vi "Start Acquisition and Logging.vi"(8 "error in (no error)":errorcluster caption="错误输入（无错误）", 11 "Acquisition and Logging Configuration":T1={"Samples per Read"=100, "Number of Reads to Save"=20, "Number of Channels"=4, "Channel Scale Array"=[1.0, 1.0, 1.0, 1.0], "Channel Names"=["Mod1\\AI0", "Mod1\\AI1", "Mod1\\AI2", "Mod1\\AI3"], "Trigger - RMS Value"=0.9999999999999994, "Trigger - Channel"=0, "Trigger - Time (Minute)"=10, "TDMS Properties"=[], "Data File Name"="cRIO_Data", "Date Rate"=20} caption="采集与记录设置" {"Date Rate" items=["51.200 kS/s (NI 9234)"=1, "25.600 kS/s (NI 9234)"=2, "17.067 kS/s (NI 9234)"=3, "12.80 kS/s (NI 9234)"=4, "10.240 kS/s (NI 9234)"=5, "8.533 kS/s (NI 9234)"=6, "7.314 kS/s (NI 9234)"=7, "6.400 kS/s (NI 9234)"=8, "5.689 kS/s (NI 9234)"=9, "5.120 kS/s (NI 9234)"=10, "4.654 kS/s (NI 9234)"=11, "4.267 kS/s (NI 9234)"=12, "3.938 kS/s (NI 9234)"=13, "3.657 kS/s (NI 9234)"=14, "3.413 kS/s (NI 9234)"=15, "3.200 kS/s (NI 9234)"=16, "3.012 kS/s (NI 9234)"=17, "2.845 kS/s (NI 9234)"=18, "2.695 kS/s (NI 9234)"=19, "2.560 kS/s (NI 9234)"=20, "2.438 kS/s (NI 9234)"=21, "2.328 kS/s (NI 9234)"=22, "2.226 kS/s (NI 9234)"=23, "2.133 kS/s (NI 9234)"=24, "2.048 kS/s (NI 9234)"=25, "1.969 kS/s (NI 9234)"=26, "1.896 kS/s (NI 9234)"=27, "1.829 kS/s (NI 9234)"=28, "1.765 kS/s (NI 9234)"=29, "1.707 kS/s (NI 9234)"=30, "1.652 kS/s (NI 9234)"=31]}) -> (0 "error out":errorcluster caption="错误输出", 1 "Wait on IRQ Timeout?":bool caption="等待IRQ超时？", 2 "Total Buffer Size":i32 caption="全部缓冲区大小", 3 "FPGA VI Reference":T4 caption="FPGA VI引用")   [LabVIEW 2013]
uses:
  controls/FPGA VI Reference.ctl
  controls/Acquisition and Logging Configuration.ctl
  controls/TDMS Properties.ctl
  <vilib>/LabVIEW Targets/FPGA/cRIO/shared/nicrio_ModuleControls/nicrio_cRIO-9234_DataRatesRing2.ctl
  <vilib>/rvi/interface/common/niFpgaWaitOnOcc.vi
  <vilib>/FPGAPlugInAG/cRIO-9074/niLvFpga_Open_cRIO-9074.vi
  <vilib>/FPGAPlugInAG/cRIO-9074/niLvFpga_Reset_cRIO-9074.vi
  <vilib>/Utility/error.llb/Error Cluster From Error Code.vi
  <vilib>/rvi/errors/niLvFpgaAdjustHostInterfaceError.vi
  <vilib>/FPGAPlugInAG/cRIO-9074/niLvFpga_Run_cRIO-9074.vi
  <vilib>/RVI Host/nirviSupport.llb/nirviErrorClusterFromErrorCode.vi
  <vilib>/rvi/interface/nirviOpenFPGA/nirviOpenFPGA.xnode
  FPGA Bitfiles/LabVIEWFPGAWavef_FPGA_FPGAMain_vTbN89OLNVY.lvbitx
  FPGA Main.vi
  <vilib>/rvi/interface/nirviMethod/nirviMethod.xnode
  <vilib>/rvi/interface/nirviReadWriteControl/nirviReadWriteControl.xnode
  <vilib>/rvi/errors/niLvFpgaMergeErrorWithErrorCode.vi
  NiFpgaLv.dll
  <vilib>/FPGAPlugInAG/cRIO-9074/niLvFpga_ConfigureFifo_cRIO-9074.vi
  <vilib>/FPGAPlugInAG/cRIO-9074/niLvFpga_StartFifo_cRIO-9074.vi
  <vilib>/rvi/interface/nirviMethod/StockFPGA_InlinedMethodWaitForSingleIRQ.vi
  <vilib>/FPGAPlugInAG/cRIO-9074/niLvFpga_WaitOnIrq_cRIO-9074.vi
  <vilib>/FPGAPlugInAG/cRIO-9074/niLvFpga_AcknowledgeIrq_cRIO-9074.vi
panel:
  # "通道"
  # "保存"
  # "采样"
  # "触发"
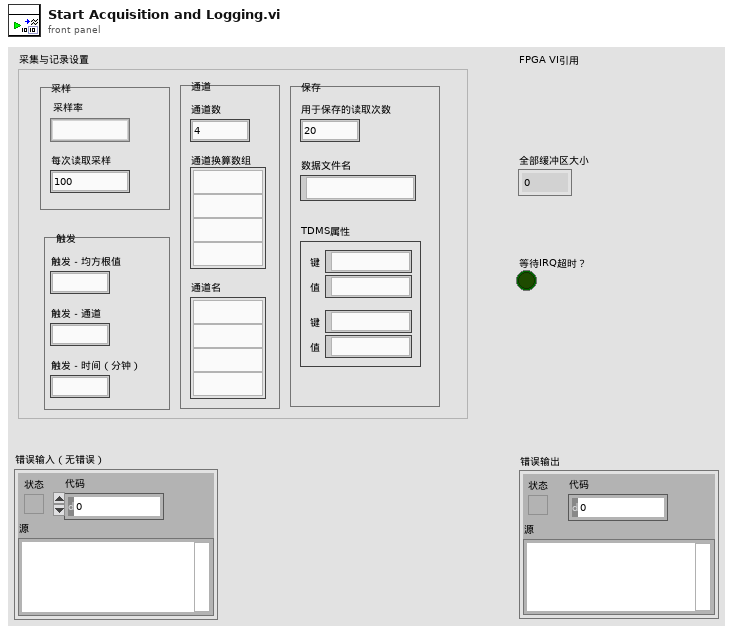
[diagram p1: front panel]
types:
  T1 = typedef "Acquisition and Logging Configuration.ctl" = cluster{"Samples per Read":i32, "Number of Reads to Save":i32, "Number of Channels":i32, "Channel Scale Array":fxp<+,24,12>[], "Channel Names":string[], "Trigger - RMS Value":dbl, "Trigger - Channel":i32, "Trigger - Time (Minute)":i32, "TDMS Properties":T2[], "Data File Name":string, "Date Rate":T3}
  T2 = typedef "TDMS Properties.ctl" = cluster{"Name":string, "Value":string}
  T3 = typedef "nicrio_cRIO-9234_DataRatesRing2.ctl" = u16
  T4 = typedef "FPGA VI Reference.ctl" = refnum<k20>
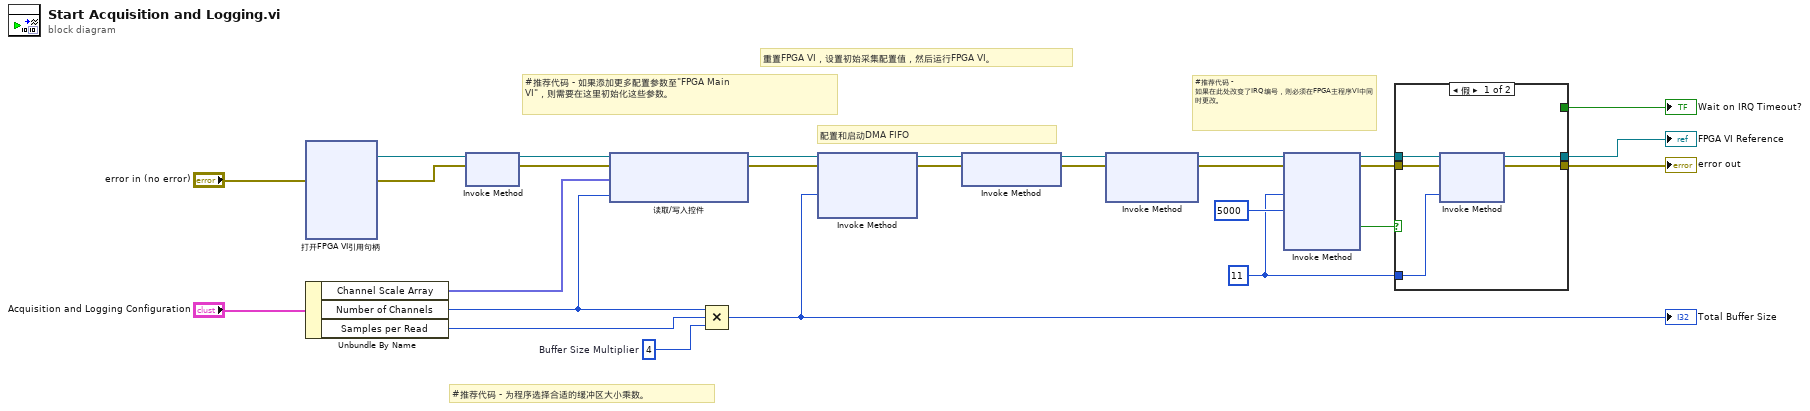
[diagram p0: block diagram]
diagram:
  w8 = 11
  w9 = u32 4  # Buffer Size Multiplier
  # "#推荐代码 - 如果在此处改变了IRQ编号，则必须在FPGA主程序VI中同时更改。"
  # "#推荐代码 - 为程序选择合适的缓冲区大小乘数。"
  # "配置和启动DMA FIFO"
  # "#推荐代码 - 如果添加更多配置参数至\"FPGA Main VI\"，则需要在这里初始化这些参数。"
  # "重置FPGA VI，设置初始采集配置值，然后运行FPGA VI。"
  n1 = xnode "打开FPGA VI引用句柄"("错误输入"="error in (no error)") -> ("FPGA VI引用输出"=w4:refnum<k20>, "错误输出"=w5:errorcluster)  [unwired: 1 in]
  n2 = Unbundle By Name("Acquisition and Logging Configuration") -> ("Channel Scale Array"=w1:fxp<+,24,12>[], "Number of Channels"=w2:i32, "Samples per Read"=w11:i32)
  n3 = xnode "Invoke Method"("FPGA VI引用输入"=w4, "错误输入"=w5) -> ("FPGA VI引用输出"=w25:refnum<k20>, "错误输出"=w24:errorcluster)
  n4 = xnode "读取/写入控件"("FPGA VI引用输入"=w25, "错误输入"=w24, "Channel Scale Array"=w1, "Number of Channels"=w2) -> ("FPGA VI引用输出"=w13:refnum<k20>, "错误输出"=w12:errorcluster)
  n5 = Compound Arithmetic op=MULTIPLY(w2, w11, w9) -> (w10:u32)
  "Total Buffer Size" <- w10
  n6 = xnode "Invoke Method"("FPGA VI引用输入"=w13, "错误输入"=w12, "请求的深度"=w10) -> ("FPGA VI引用输出"=w16:refnum<k20>, "错误输出"=w17:errorcluster)  [unwired: 1 out]
  n7 = xnode "Invoke Method"("FPGA VI引用输入"=w16, "错误输入"=w17) -> ("FPGA VI引用输出"=w14:refnum<k20>, "错误输出"=w15:errorcluster)
  n8 = xnode "Invoke Method"("FPGA VI引用输入"=w14, "错误输入"=w15) -> ("FPGA VI引用输出"=w26:refnum<k20>, "错误输出"=w27:errorcluster)  [unwired: 1 in]
  n9 = xnode "Invoke Method"("FPGA VI引用输入"=w26, "错误输入"=w27, "IRQ编号"=w8, "超时(ms)"=5000 ("Timeout (ms)")) -> ("FPGA VI引用输出"=w18:refnum<k20>, "错误输出"=w19:errorcluster, "超时"=w21:bool)  [unwired: 1 out]
  n10 = case shown="假" w21 {
    selector: w21 -> [_ w33]
    tunnel: w18 -> [w32 w34]
    tunnel: w19 -> [w31 w35]
    tunnel: [w30 w35] -> w22
    tunnel: w8 -> [w29 _]
    tunnel: [_ w33] -> w23
    tunnel: [w28 w34] -> w7
    frame False {
      n11 = xnode "Invoke Method"("FPGA VI引用输入"=w32, "错误输入"=w31, "IRQ编号"=w29) -> ("FPGA VI引用输出"=w28:refnum<k20>, "错误输出"=w30:errorcluster)
    }
    frame True {
    }
  }
  "Wait on IRQ Timeout?" <- w23
  "error out" <- w22
  "FPGA VI Reference" <- w7
